vi "Apply Torque to Drivebase.vi"(9 "Gear Ratio (out/in)":dbl=0.05, 10 "Robot Characterization":T1={"Total Mass"=68.0388555, "Wheel Friction"=1.0, "Wheel Diameter"=0.15239999999999998}, 11 "Motor Torque":dbl[unit]=5.0) -> (0 "slip":bool, 2 "Motor Angular accel":dbl[unit], 3 "Robot Accel":dbl[unit])   [LabVIEW 2019]
panel:
  out "F friction":dbl[unit]
  out "F motors":dbl[unit]
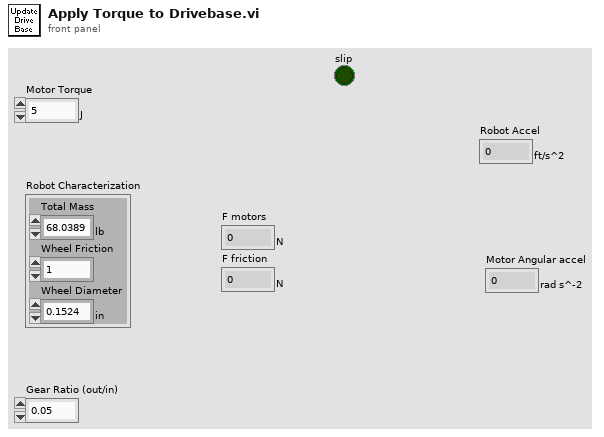
[diagram p1: front panel]
types:
  T1 = cluster{"Total Mass":dbl[unit], "Wheel Friction":dbl, "Wheel Diameter":dbl[unit]}
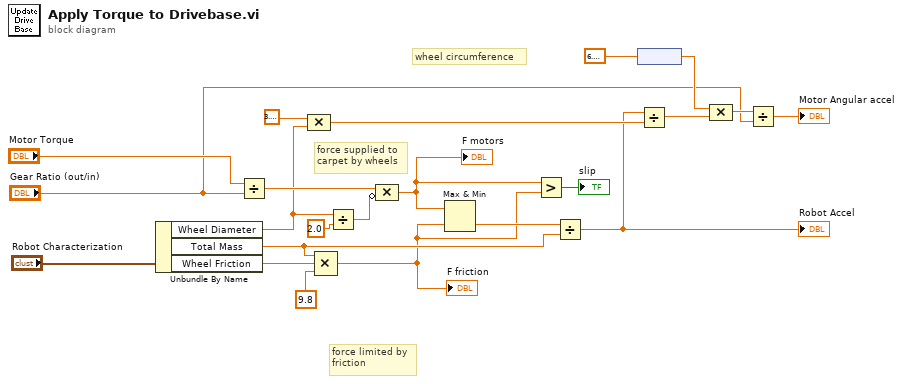
[diagram p0: block diagram]
diagram:
  # "wheel circumference"
  # "force supplied to\ncarpet by wheels"
  # "force limited by\nfriction"
  n1 = Unbundle By Name("Robot Characterization") -> ("Wheel Diameter"=w13:dbl[unit], "Total Mass"=w14:dbl[unit], "Wheel Friction"=w20:dbl)
  n2 = Divide(x="Motor Torque", y="Gear Ratio (out/in)") -> (x/y=w18:dbl[unit])
  n3 = Compound Arithmetic op=MULTIPLY(3.141592653589793, w13) -> (w11:dbl[unit])
  n4 = Compound Arithmetic op=MULTIPLY(w14, w20, dbl[unit] 9.8 ("value")) -> (w2:dbl[unit])
  "F friction" <- w2
  n5 = Divide(x=w13, y=2.0) -> (x/y=w17:dbl[unit])
  n6 = Compound Arithmetic op=MULTIPLY(w18, invert w17) -> (w3:dbl[unit])
  "F motors" <- w3
  n7 = Max & Min(x=w3, y=w2) -> (min(x,y)=w15:dbl[unit])  [unwired: 1 out]
  n8 = Greater?(x=w3, y=w2) -> (0:→"slip":bool)
  n9 = Divide(x=w15, y=w14) -> (x/y=w10:dbl[unit])
  "Robot Accel" <- w10
  n10 = node(6.283185307179586) -> (w7:dbl[unit])
  n11 = Divide(x=w10, y=w11) -> (x/y=w9:dbl[unit])
  n12 = Compound Arithmetic op=MULTIPLY(w7, w9) -> (w6:dbl[unit])
  n13 = Divide(x=w6, y="Gear Ratio (out/in)") -> (x/y=→"Motor Angular accel":dbl[unit])
